vi "AddLoadModules.vi"(8 "error in":errorcluster, 11 "Config in":T1) -> (0 "error out":errorcluster, 3 "Config out":T1)   [LabVIEW 2020]
uses:
  <vilib>/WebServerConfig/Config.ctl
  <vilib>/WebServerConfig/Server.ctl
  <vilib>/WebServerConfig/Alias.ctl
  <vilib>/WebServerConfig/ErrorDocument.ctl
  <vilib>/WebServerConfig/Action.ctl
  <vilib>/WebServerConfig/Redirect.ctl
  <vilib>/WebServerConfig/Interface.ctl
  <vilib>/WebServerConfig/AddHandler.ctl
  <vilib>/WebServerConfig/SSL.ctl
  <vilib>/WebServerConfig/CustomLog.ctl
  <vilib>/WebServerConfig/LoadModule.ctl
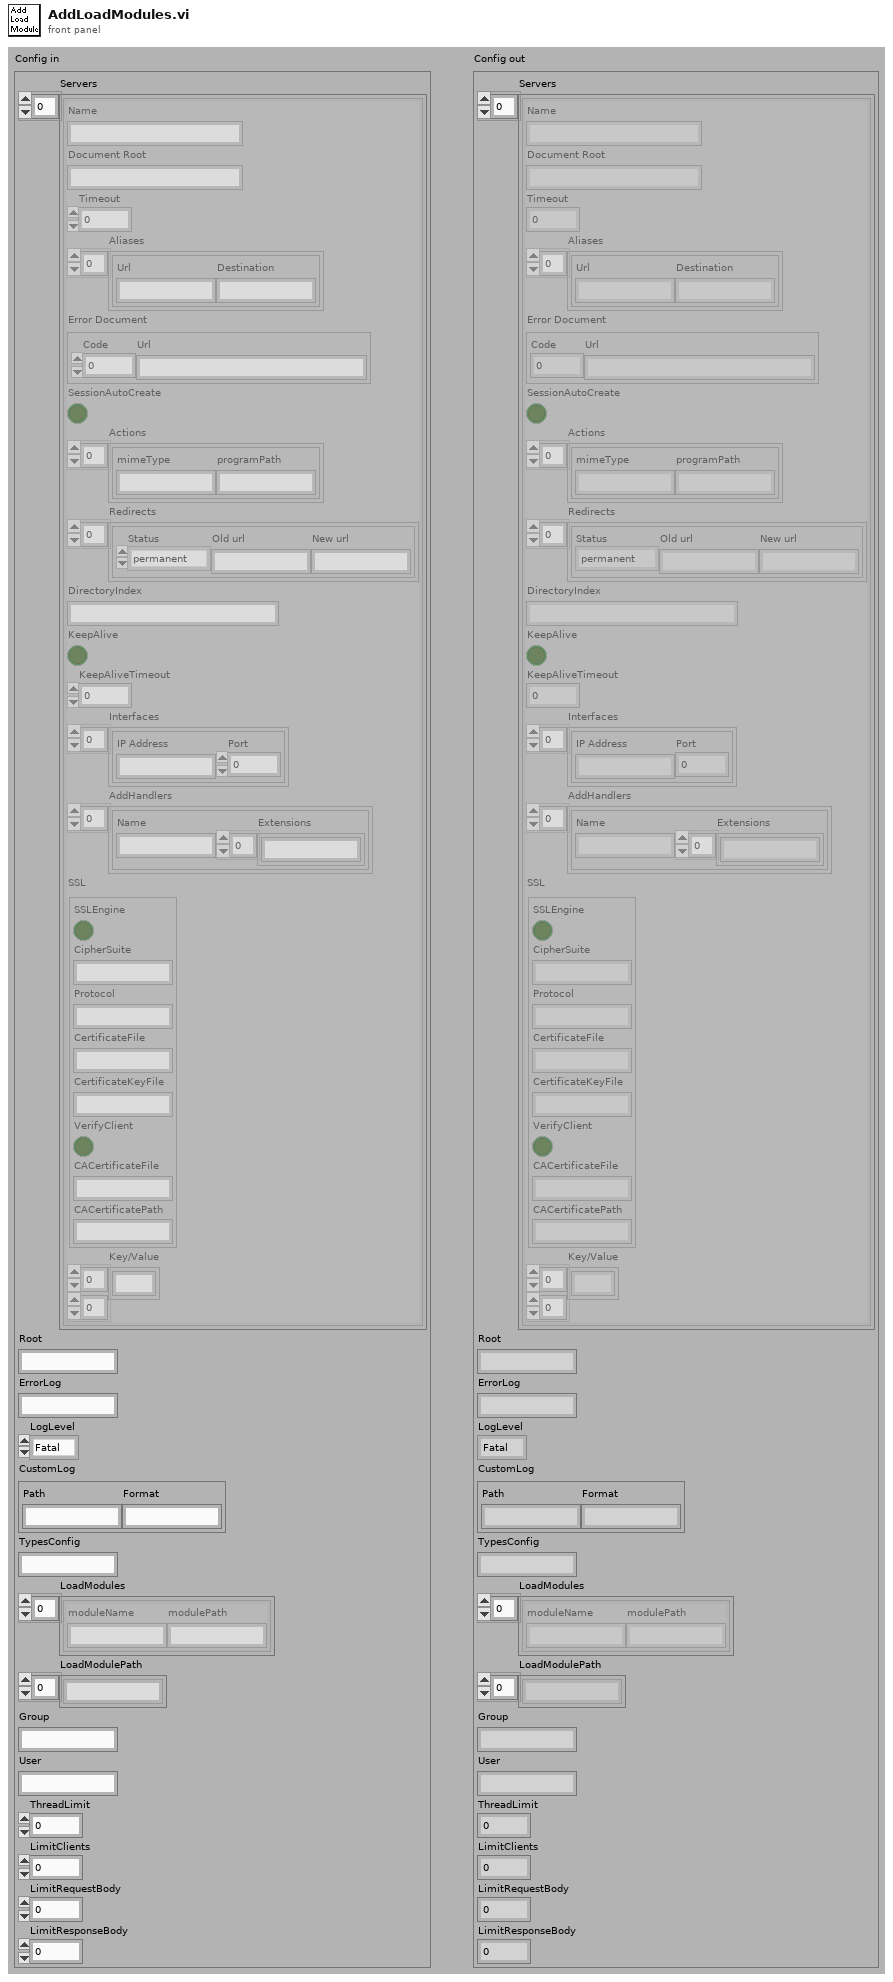
[diagram p1: front panel]
types:
  T1 = typedef "Config.ctl" = cluster{"Servers":T2[], "Root":string, "ErrorLog":string, "LogLevel":enum16{"Fatal", "Error", "Warn", "Info", "Debug", "5", "6", "7", "8", "Verbose"}, "CustomLog":T10, "TypesConfig":string, "LoadModules":T11[], "LoadModulePath":string[], "Group":string, "User":string, "ThreadLimit":u32, "LimitClients":u32, "LimitRequestBody":u32, "LimitResponseBody":u32}
  T2 = typedef "Server.ctl" = cluster{"Name":string, "Document Root":string, "Timeout":u32, "Aliases":T3[], "Error Document":T4, "SessionAutoCreate":bool, "Actions":T5[], "Redirects":T6[], "DirectoryIndex":string, "KeepAlive":bool, "KeepAliveTimeout":u32, "Interfaces":T7[], "AddHandlers":T8[], "SSL":T9, "Key/Value":string[][]}
  T3 = typedef "Alias.ctl" = cluster{"Url":string, "Destination":string}
  T4 = typedef "ErrorDocument.ctl" = cluster{"Code":u16, "Url":string}
  T5 = typedef "Action.ctl" = cluster{"mimeType":string, "programPath":string}
  T6 = typedef "Redirect.ctl" = cluster{"Status":enum16{"permanent", "temp", "seeother", "gone"}, "Old url":string, "New url":string}
  T7 = typedef "Interface.ctl" = cluster{"IP Address":string, "Port":u16}
  T8 = typedef "AddHandler.ctl" = cluster{"Name":string, "Extensions":string[]}
  T9 = typedef "SSL.ctl" = cluster{"SSLEngine":bool, "CipherSuite":string, "Protocol":string, "CertificateFile":string, "CertificateKeyFile":string, "VerifyClient":bool, "CACertificateFile":string, "CACertificatePath":string}
  T10 = typedef "CustomLog.ctl" = cluster{"Path":string, "Format":string}
  T11 = typedef "LoadModule.ctl" = cluster{"moduleName":string, "modulePath":string}
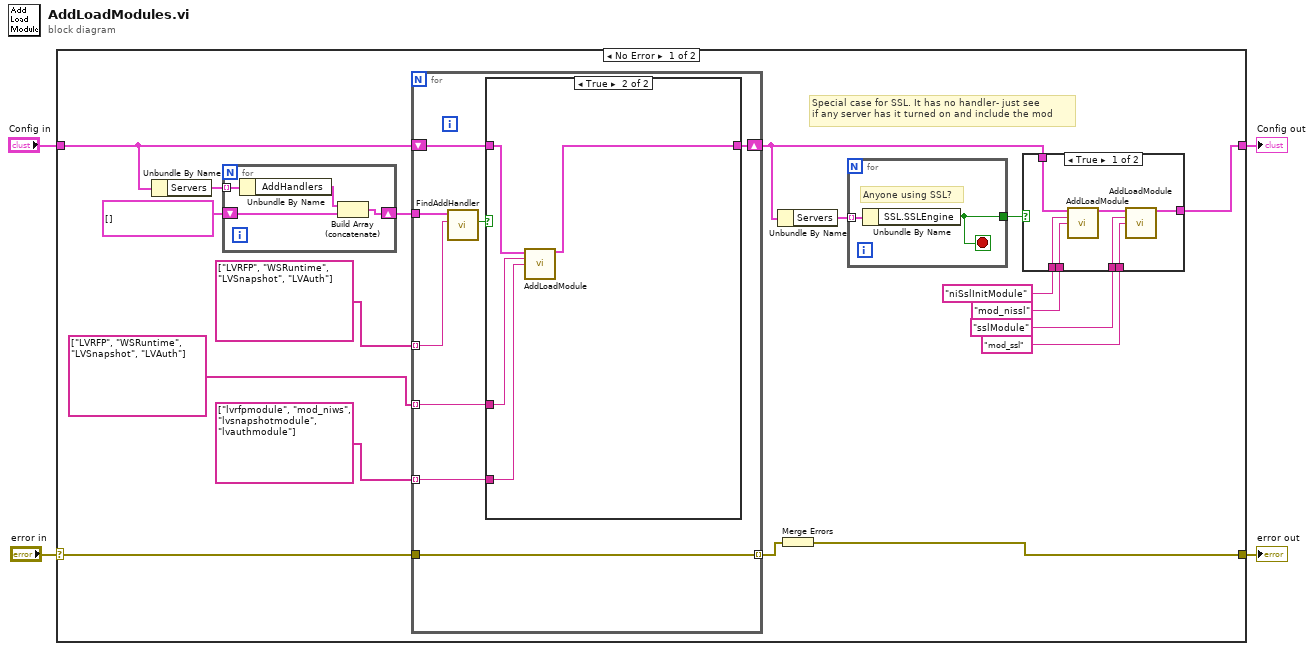
[diagram p0: block diagram]
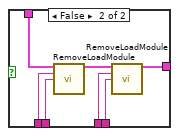
[diagram p2: hidden frame]
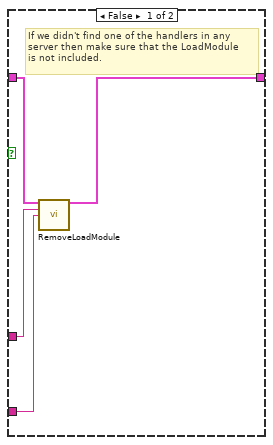
[diagram p3: hidden frame]
diagram:
  n1 = case shown="No Error" "error in" {
    selector: "error in" -> [w17 w60]
    tunnel: [w16 w60] -> w3
    tunnel: [w11 w59] -> w1
    tunnel: "Config in" -> [w20 w59]
    frame No Error {
      # "Special case for SSL. It has no handler- just see\nif any server has it turned on and include the mod"
      n2 = Unbundle By Name(w20) -> ("Servers"=w22:T2[])
      n3 = for {
        tunnel: w22 -> [w58] mode=indexing
        shift-right: [w56] -> w19
        shift-left: T8[] [] -> [w55]
        n4 = Unbundle By Name(w58) -> ("AddHandlers"=w57:T8[])
        n5 = Build Array (concatenate)(w57, w55) -> (w56:T8[])
      }
      n6 = for {
        tunnel: string[] ["LVRFP", "WSRuntime", "LVSnapshot", "LVAuth"] ("Handlers") -> [w42] mode=indexing
        tunnel: w19 -> [w44]
        shift-right: [w45] -> w7
        shift-left: w20 -> [w46]
        tunnel: w17 -> [w40]
        tunnel: [w40] -> w15 mode=indexing
        tunnel: string[] ["LVRFP", "WSRuntime", "LVSnapshot", "LVAuth"] ("Handlers") -> [w41] mode=indexing
        tunnel: string[] ["lvrfpmodule", "mod_niws", "lvsnapshotmodule", "lvauthmodule"] ("Handlers") -> [w43] mode=indexing
        n7 = call <vilib>:"FindAddHandler.vi"("Name"=w42, "AddHandlers"=w44) -> ("Found"=w39:bool)  [unwired: 2 in, 7 out]
        n8 = case shown="True" w39 {
          tunnel: w46 -> [w50 w54]
          tunnel: [w47 w53] -> w45
          tunnel: w41 -> [w49 w52]
          tunnel: w43 -> [w48 w51]
          frame False {
            # "If we didn't find one of the handlers in any\nserver then make sure that the LoadModule\nis not included."
            n9 = call <vilib>:"RemoveLoadModule.vi"("Config in"=w50, "Name"=w49, "Path"=w48) -> ("Config out"=w47:T1)  [unwired: 1 in, 11 out]
          }
          frame True {
            n10 = call <vilib>:"AddLoadModule.vi"("Config in"=w54, "name"=w52, "path"=w51) -> ("Config out"=w53:T1)  [unwired: 1 in, 11 out]
          }
        }
      }
      n11 = Unbundle By Name(w7) -> ("Servers"=w12:T2[])
      n12 = Merge Errors(w15) -> (w16:errorcluster)
      n13 = for {
        tunnel: w12 -> [w38] mode=indexing
        tunnel: [w37] -> w8
        stop <- w37 stop-if-true
        # "Anyone using SSL?"
        n14 = Unbundle By Name(w38) -> ("SSL.SSLEngine"=w37:bool)
      }
      n15 = case shown="True" w8 {
        tunnel: [w23 w30] -> w11
        tunnel: "sslModule" -> [w29 w36]
        tunnel: "mod_ssl" -> [w28 w35]
        tunnel: w7 -> [w26 w34]
        tunnel: "niSslInitModule" -> [w24 w32]
        tunnel: "mod_nissl" -> [w25 w31]
        frame True {
          n16 = call <vilib>:"AddLoadModule.vi"("Config in"=w26, "name"=w24, "path"=w25) -> ("Config out"=w27:T1)  [unwired: 1 in, 11 out]
          n17 = call <vilib>:"AddLoadModule.vi"("Config in"=w27, "name"=w29, "path"=w28) -> ("Config out"=w23:T1)  [unwired: 1 in, 11 out]
        }
        frame False {
          n18 = call <vilib>:"RemoveLoadModule.vi"("Config in"=w34, "Name"=w32, "Path"=w31) -> ("Config out"=w33:T1)  [unwired: 12 out]
          n19 = call <vilib>:"RemoveLoadModule.vi"("Config in"=w33, "Name"=w36, "Path"=w35) -> ("Config out"=w30:T1)  [unwired: 12 out]
        }
      }
    }
    frame Error {
    }
  }
  "error out" <- w3
  "Config out" <- w1
